vi "Connect Route.vi"(6 "Mux Index":i32, 8 "error in (no error)":errorcluster, 9 "Output":i32, 10 "Input":i32, 11 "MuxAPI in":refnum<class "MuxAPI.lvclass">) -> (0 "error out":errorcluster, 2 "Routes":cluster{"Mux Route":i32[]}[](array[cluster]), 3 "MuxAPI out":refnum<class "MuxAPI.lvclass">)   [LabVIEW 2022 SP3, in "VideoMux.lvlib" / "MuxAPI.lvclass"]
uses:
  MuxAPI.lvclass
  MuxAPI.lvclass/MuxAPI.ctl
  MuxActor Messages/Connect Route Msg/Connect Route Msg.lvclass
  <vilib>/IlluminatedG/IG Promises/Promises/Promise/Promise.lvclass
  MuxRoute Value/MuxRoute Value.lvclass
  <vilib>/IlluminatedG/IG Promises/Promises/Future/Future.lvclass
  C:/Program Files (x86)/National Instruments/LabVIEW 2022/vi.lib/IlluminatedG/IG Promises/Promises/Value/Value.lvclass
  C:/dev/illuminatedg/TouchControl/VideoMux/MuxRoute Value/MuxRoute Value.lvclass
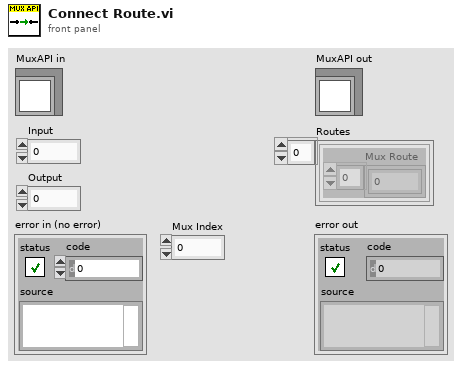
[diagram p1: front panel]
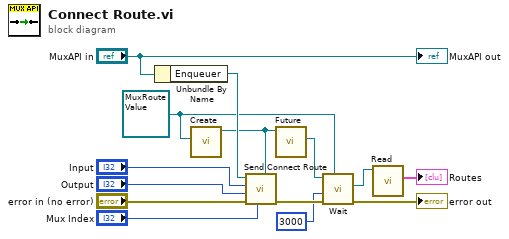
[diagram p0: block diagram]
diagram:
  w10 = refnum<class "MuxRoute Value.lvclass"> refnum ("VideoMux.lvlib:MuxRoute Value.lvclass")
  n1 = Unbundle By Name("MuxAPI in") -> ("Enqueuer"=w12:refnum<class "Message Enqueuer.lvclass">)
  n2 = call <vilib>:"Create.vi"("Result Type"=w10) -> ("Promise"=w11:refnum<class "Promise.lvclass">)  [unwired: 9 in, 1 out]
  n3 = call "Send Connect Route.vi"("Promise in"=w11, "Mux Index"="Mux Index", "error in (no error)"="error in (no error)", "Output"="Output", "Input"="Input", "Message Enqueuer"=w12) -> ("error out"=w6:errorcluster)  [unwired: 4 in, 1 out]
  n4 = call <vilib>:"Future.vi"("Promise in"=w11) -> ("Future"=w2:refnum<class "Future.lvclass">)  [unwired: 9 in, 1 out]
  n5 = call <vilib>:"Wait.vi"("Result Type"=w10, "error in (no error)"=w6, "Timeout mS (-1)"=3000, "Future in"=w2) -> ("error out"=→"error out":errorcluster, "Result"=w4:refnum<class "MuxRoute Value.lvclass">)  [unwired: 6 in]
  n6 = call "Read.vi"("MuxRoute Value in"=w4) -> ("Muxes"=→"Routes":cluster{"Mux Route":i32[]}[])  [unwired: 10 in]
  "MuxAPI out" <- "MuxAPI in"
